vi "ztscopeM Vertical.vi"(0 "Instrument Handle In":i32, 1 "Coupling":i32(ring)=1 items=["AC", "DC", "ACLFR"], 2 "Impedance":dbl(ring)=50.0 items=["50 Ohm"=50.0, "1 MOhm"=1000000.0], 5 "Channel":i32(ring) items=["Input Channel 1", "Input Channel 2", "Input Channel 3", "Input Channel 4"], 7 "Range":dbl=10.0, 9 "Offset":dbl, 11 "error in":errorcluster, 12 "Lowpass Filter":i32(ring) items=["Bypass", "Lowpass"], 13 "Attenuation":dbl=1.0) -> (4 "Instrument Handle Out":i32, 15 "error out":errorcluster)   [LabVIEW 2013]
doc: "Configure the vertical settings for the selected channel"
uses:
  ztscopeM.dll
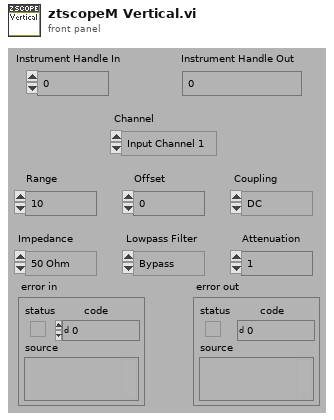
[diagram p1: front panel]
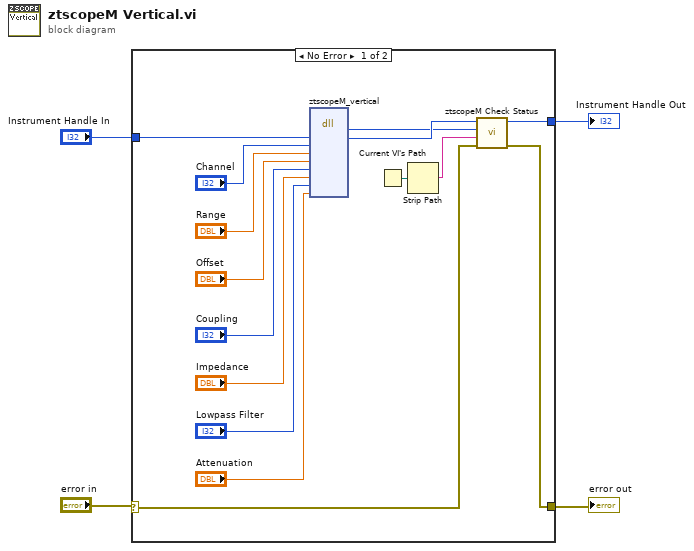
[diagram p0: block diagram]
diagram:
  n1 = case shown="No Error" "error in" {
    selector: "error in" -> [w7 w20]
    tunnel: [w6 w20] -> w2
    tunnel: "Instrument Handle In" -> [w19 w21]
    tunnel: [w5 w21] -> w3
    frame No Error {
      n2 = dll-call lib="C:/Program Files/National Instruments/instr.lib/ztscopem/ztscopeM.dll" fn="ztscopeM_vertical"("instrumentHandle"=w19, "channel"="Channel", "range"="Range", "offset"="Offset", "coupling"="Coupling", "impedance"="Impedance", "lowpassFilter"="Lowpass Filter", "attenuation"="Attenuation") -> (w8:i32, "instrumentHandle"=w9:i32)  [unwired: 10 in, 2 out]
      n3 = Current VI's Path() -> (path=w11:path)
      n4 = Strip Path(path=w11) -> (name=w10:string)  [unwired: 1 out]
      n5 = call "ztscopeM Check Status.vi"("error in"=w7, "name of VI"=w10, "status"=w8, "instrument handle in"=w9) -> ("error out"=w6:errorcluster, "instrument handle out"=w5:i32)  [unwired: 2 in]
    }
    frame Error {
    }
  }
  "Instrument Handle Out" <- w3
  "error out" <- w2
